vi "Chart Demo with Limits.vi"() -> ()   [LabVIEW 2019]
uses:
  <vilib>/numeric/Random Number (Range) DBL.vi
panel:
  in  "Stop":bool
  out "Waveform Chart":dbl[][](graph)
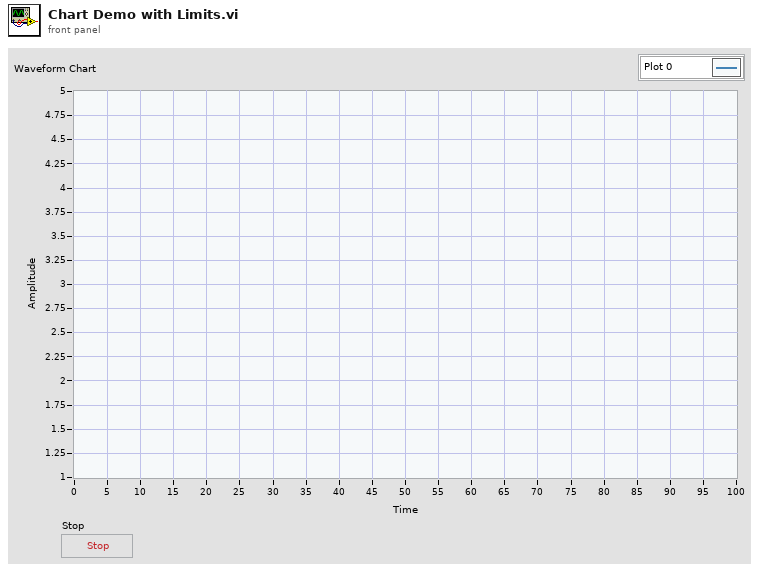
[diagram p1: front panel]
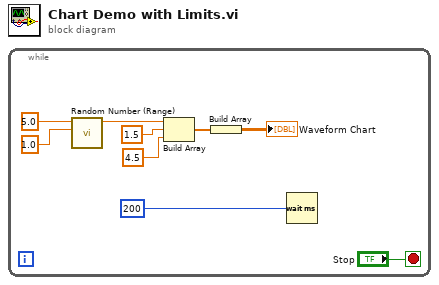
[diagram p0: block diagram]
diagram:
  n1 = while {
    stop <- "Stop" stop-if-true
    n2 = call-poly <vilib>:"Random Number (Range).vi"("lower bound (0)"=1.0, "upper bound (100)"=5.0) -> ("number"=w1:dbl)  [unwired: 9 in]
    n3 = Build Array(w1, 1.5 ("element"), 4.5 ("element")) -> (w7:dbl[])
    n4 = Build Array(w7) -> (→"Waveform Chart":dbl[][])
    n5 = Wait (ms)(milliseconds to wait=u32 200) -> ()  [unwired: 1 out]
  }
